vi "Firmware Manager.vi"() -> ()   [LabVIEW 2018]
uses:
  Type Defs/Firmware Action.ctl
  Type Defs/State Machine.ctl
panel:
  out "Wait":bool
  out "Error Out":errorcluster
  in  "Error In":errorcluster
  in  "Exit":bool
  in  "Start":bool
  out "Description":string
  in  "Firmware Backup Folder":path
  out "Messages":string
  in  "FW Action":T1
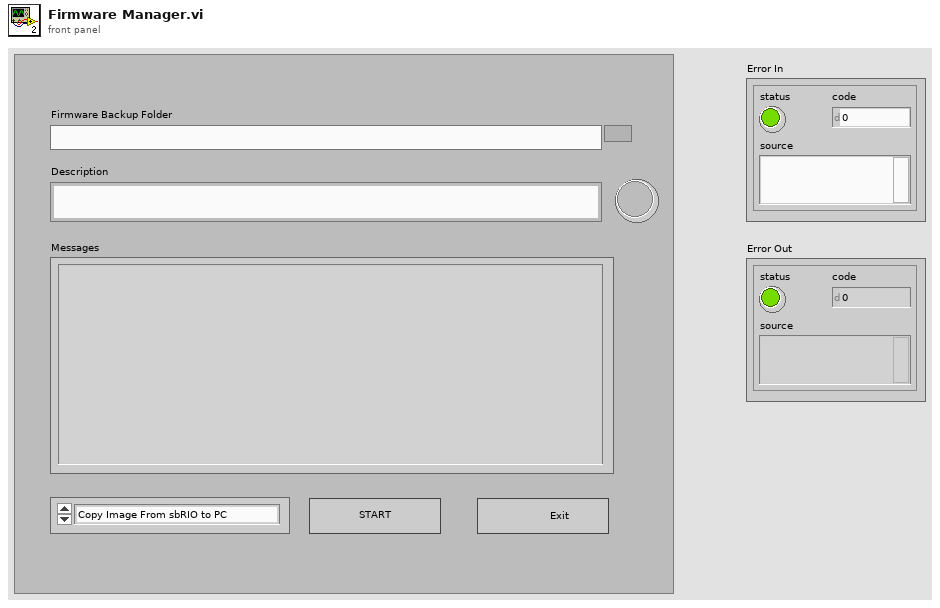
[diagram p1: front panel]
types:
  T1 = typedef "Firmware Action.ctl" = enum16{"Copy Image From sbRIO to PC", "Update Firmware From PC"}
  T2 = enum8{"Enabled", "Disabled", "Disabled and Grayed Out"}
  T3 = typedef "State Machine.ctl" = enum16{"Init", "Case 0", "Case 1", "Case 2", "Case 3", "Case 4", "Case 5", "Case 6", "Case 7", "Case 8", "Case 9", "Case 10", "Error", "Exit"}
  T4 = cluster{"Model":string, "MAC Address":string, "Hostname":string}
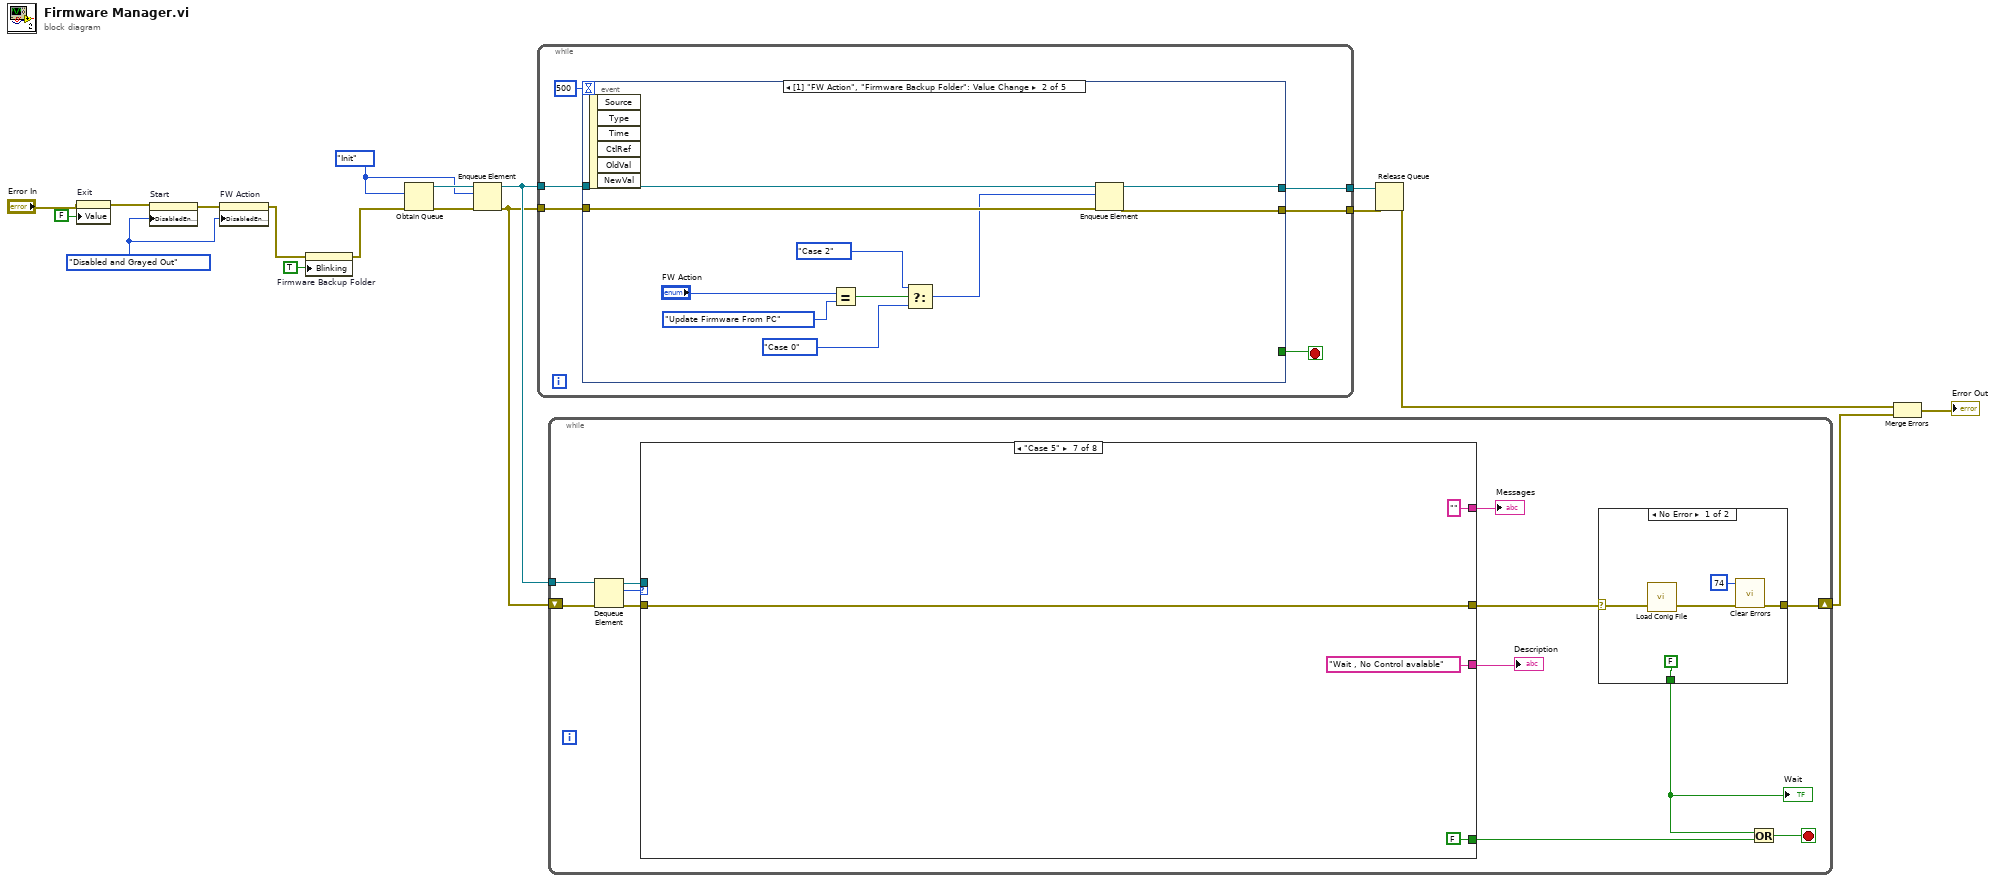
[diagram p0: block diagram]
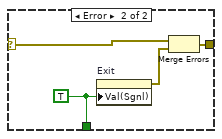
[diagram p2: hidden frame]
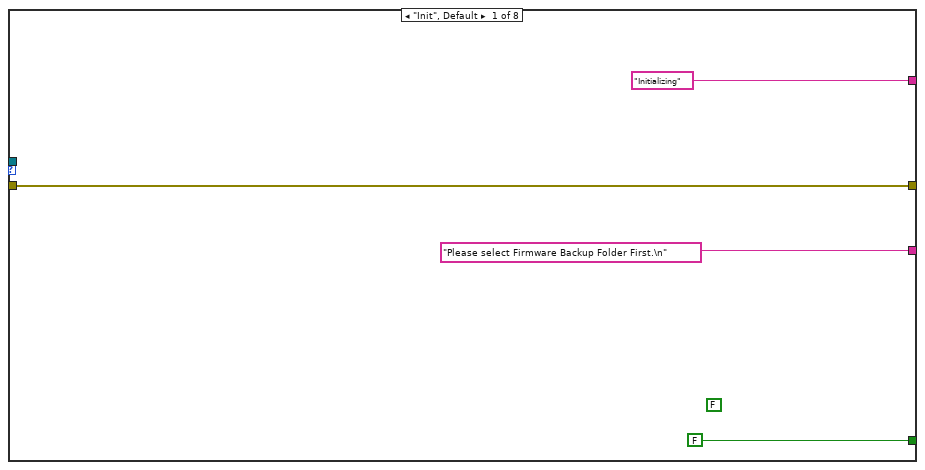
[diagram p3: hidden frame]
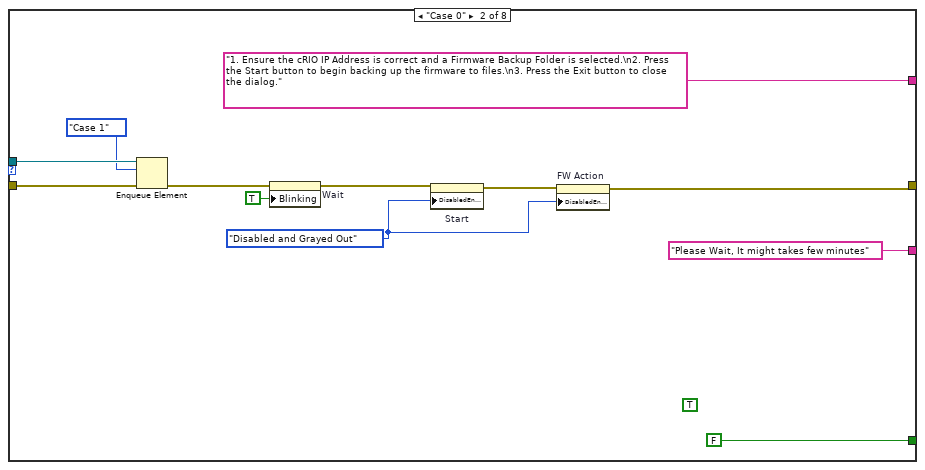
[diagram p4: hidden frame]
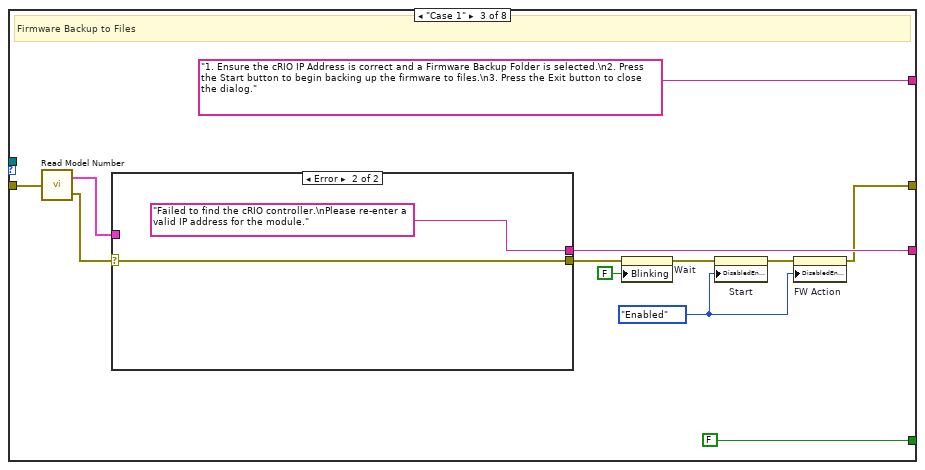
[diagram p5: hidden frame]
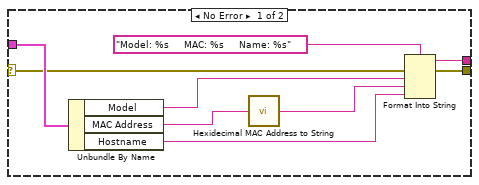
[diagram p6: hidden frame]
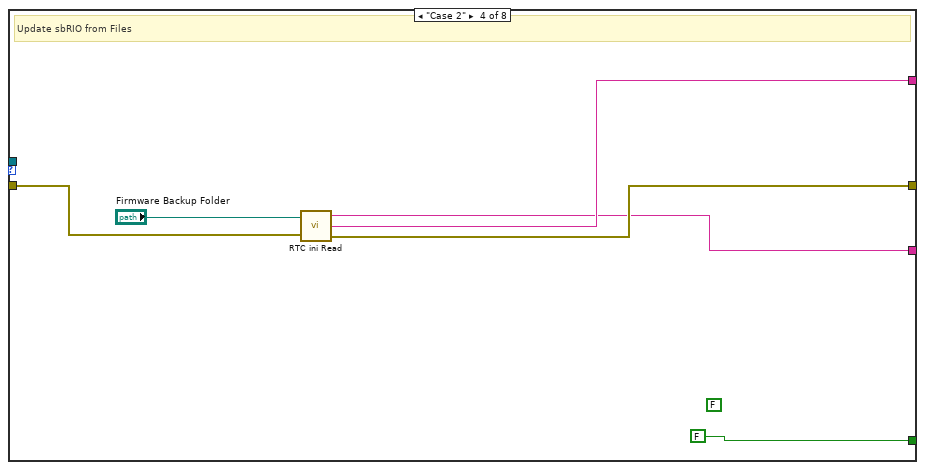
[diagram p7: hidden frame]
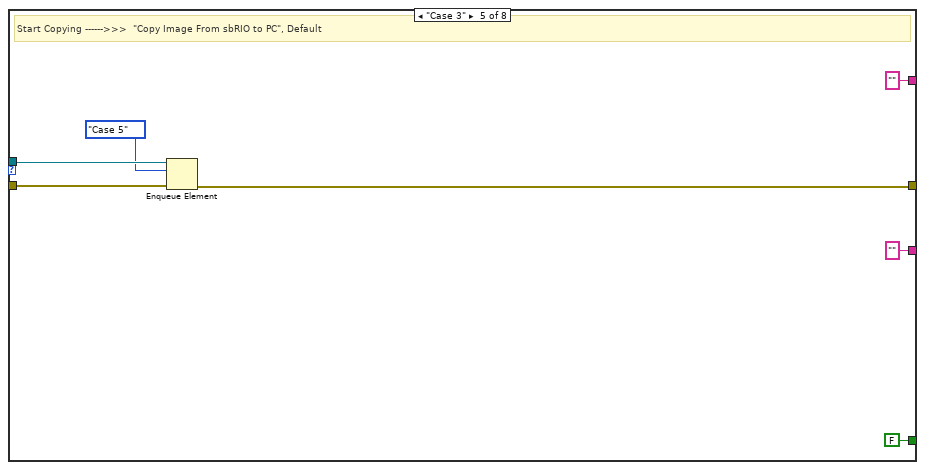
[diagram p8: hidden frame]
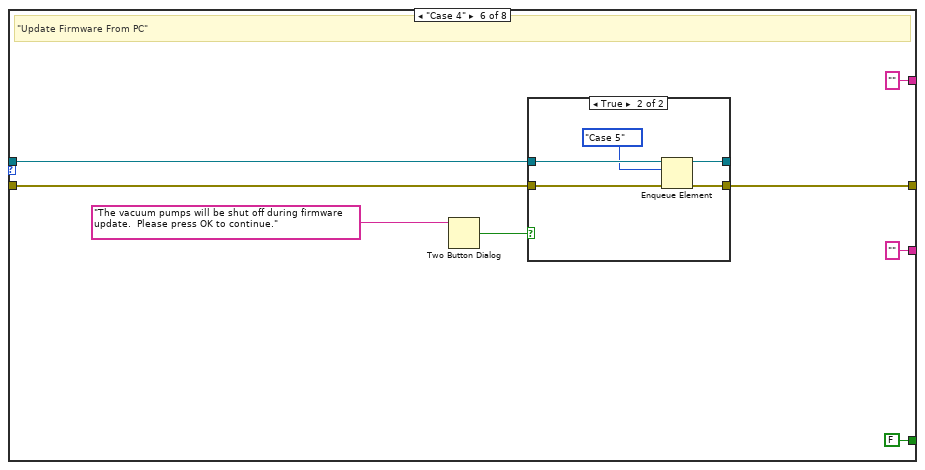
[diagram p9: hidden frame]
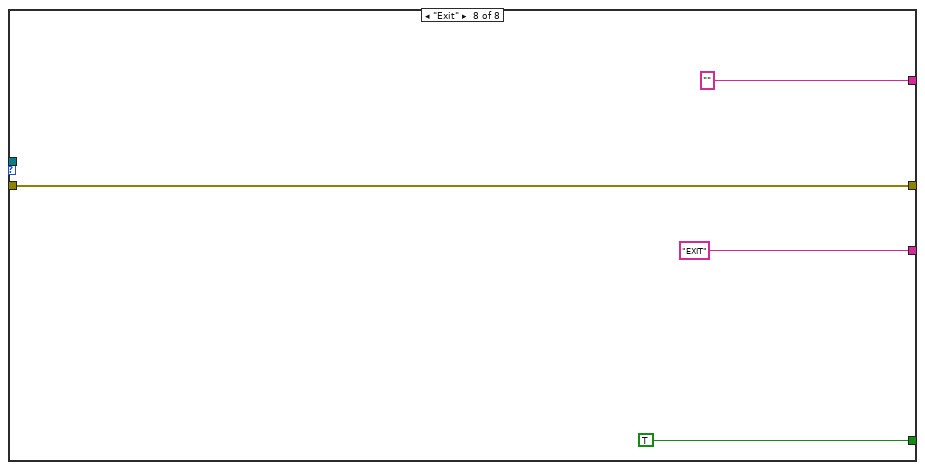
[diagram p11: hidden frame]
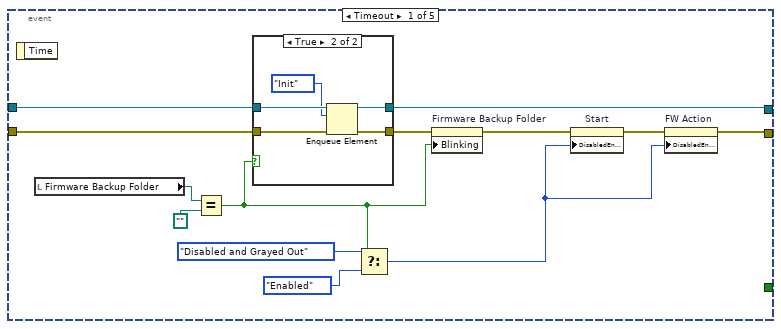
[diagram p12: hidden frame]
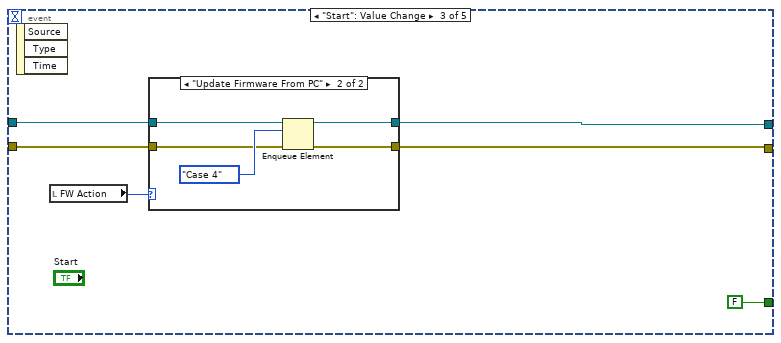
[diagram p14: hidden frame]
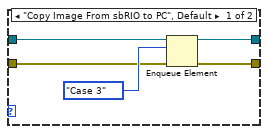
[diagram p15: hidden frame]
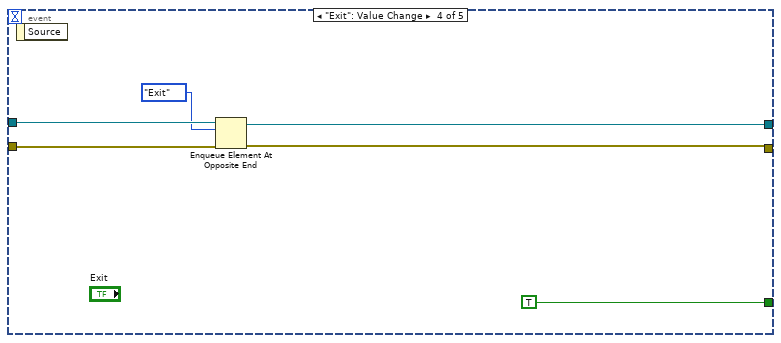
[diagram p16: hidden frame]
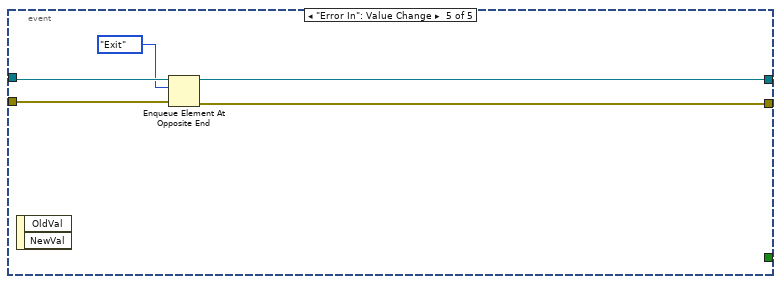
[diagram p17: hidden frame]
diagram:
  w4 = T2."Disabled and Grayed Out" ("Disabled")
  w16 = State_Machine."Init" ("Enum")
  n1 = property on="Exit" class="Bool (strict)"(error in="Error In", "Value"=FALSE ("Exit")) -> (error out=w6:errorcluster)  [unwired: 1 in, 1 out]
  n2 = property on="Start" class="Bool"(error in=w6, "DisabledEnum"=w4) -> (error out=w5:errorcluster)  [unwired: 1 in, 1 out]
  n3 = property on="FW Action" class="Enum (strict)"(error in=w5, "DisabledEnum"=w4) -> (error out=w3:errorcluster)  [unwired: 1 in, 1 out]
  n4 = property on="Firmware Backup Folder" class="Path"(error in=w3, "Blinking"=TRUE) -> (error out=w2:errorcluster)  [unwired: 1 in, 1 out]
  n5 = Obtain Queue(element data type=w16, error in (no error)=w2) -> (queue out=w18:refnum<queue>, error out=w17:errorcluster)  [unwired: 3 in, 1 out]
  n6 = Enqueue Element(queue=w18, element=w16, error in (no error)=w17) -> (queue out=w15:refnum<queue>, error out=w14:errorcluster)  [unwired: 1 in, 1 out]
  n7 = while {
    tunnel: w15 -> [w23]
    tunnel: w14 -> [w24]
    tunnel: [w20] -> w13
    tunnel: [w19] -> w10
    stop <- w22 stop-if-true
    n8 = event shown="[1] \"FW Action\", \"Firmware Backup Folder\": Value Change" {
      selector: _ -> [_ _ _ _ _]
      dyn-events: _ -> [_ _ _ _ _]
      timeout: 500 -> [_ _ _ _ _]
      tunnel: w24 -> [w28 w54 w58 w75 w81]
      tunnel: w23 -> [w27 w53 w57 w74 w80]
      tunnel: [_ _ FALSE TRUE _] -> w22
      tunnel: [w26 w52 w56 w71 w78] -> w19
      tunnel: [w34 w51 w55 w72 w77] -> w20
      event Timeout {
        n9 = event-data() -> ()  [unwired: 1 in, 1 out]
        n10 = local read "Firmware Backup Folder"() -> (w30:path)
        n11 = Equal?(x=w30, y=path "") -> (x = y?=w29:bool)
        n12 = case shown="True" w29 {
          tunnel: w28 -> [w38 w42]
          tunnel: w27 -> [w39 w44]
          tunnel: [w38 w41] -> w25
          tunnel: [w39 w40] -> w26
          frame False {
          }
          frame True {
            n13 = Enqueue Element(queue=w44, element=State_Machine."Init" ("Enum"), error in (no error)=w42) -> (queue out=w40:refnum<queue>, error out=w41:errorcluster)  [unwired: 1 in, 1 out]
          }
        }
        n14 = Select(t=T2."Disabled and Grayed Out" ("Disabled"), s=w29, f=T2."Enabled" ("Disabled")) -> (s? t:f=w32:T2)
        n15 = property on="Firmware Backup Folder" class="Path"(error in=w25, "Blinking"=w29) -> (error out=w31:errorcluster)  [unwired: 1 in, 1 out]
        n16 = property on="Start" class="Bool"(error in=w31, "DisabledEnum"=w32) -> (error out=w33:errorcluster)  [unwired: 1 in, 1 out]
        n17 = property on="FW Action" class="Enum (strict)"(error in=w33, "DisabledEnum"=w32) -> (error out=w34:errorcluster)  [unwired: 1 in, 1 out]
      }
      event "Firmware Backup Folder": Value Change {
        n18 = event-data() -> ()  [unwired: 1 in, 6 out]
        n19 = Equal?(x="FW Action", y=Firmware_Action."Update Firmware From PC" ("FW Action")) -> (x = y?=w48:bool)
        n20 = Select(t=State_Machine."Case 2" ("Enum"), s=w48, f=State_Machine."Case 0" ("Enum")) -> (s? t:f=w45:T3)
        n21 = Enqueue Element(queue=w53, element=w45, error in (no error)=w54) -> (queue out=w52:refnum<queue>, error out=w51:errorcluster)  [unwired: 1 in, 1 out]
      }
      event "Start": Value Change {
        n22 = event-data() -> ()  [unwired: 1 in, 3 out]
        n23 = local read "FW Action"() -> (w59:T1)
        n24 = case shown="\"Update Firmware From PC\"" w59 {
          tunnel: w58 -> [w64 w69]
          tunnel: w57 -> [w63 w68]
          tunnel: [w62 w67] -> w55
          tunnel: [w61 w66] -> w56
          frame "Copy Image From sbRIO to PC", Default {
            n25 = Enqueue Element(queue=w63, element=State_Machine."Case 3" ("Enum"), error in (no error)=w64) -> (queue out=w61:refnum<queue>, error out=w62:errorcluster)  [unwired: 1 in, 1 out]
          }
          frame "Update Firmware From PC" {
            n26 = Enqueue Element(queue=w68, element=State_Machine."Case 4" ("Enum"), error in (no error)=w69) -> (queue out=w66:refnum<queue>, error out=w67:errorcluster)  [unwired: 1 in, 1 out]
          }
        }
      }
      event "Exit": Value Change {
        n27 = event-data() -> ()  [unwired: 1 in, 1 out]
        n28 = Enqueue Element At Opposite End(queue=w74, element=State_Machine."Exit" ("Enum"), error in (no error)=w75) -> (queue out=w71:refnum<queue>, error out=w72:errorcluster)  [unwired: 1 in, 1 out]
      }
      event "Error In": Value Change {
        n29 = event-data() -> ()  [unwired: 1 in, 2 out]
        n30 = Enqueue Element At Opposite End(queue=w80, element=State_Machine."Exit" ("Enum"), error in (no error)=w81) -> (queue out=w78:refnum<queue>, error out=w77:errorcluster)  [unwired: 1 in, 1 out]
      }
    }
  }
  n31 = while {
    tunnel: w15 -> [w93]
    shift-right: [w85] -> w12
    shift-left: w14 -> [w92]
    stop <- w87 stop-if-true
    n32 = Dequeue Element(queue=w93, error in (no error)=w92) -> (queue out=w90:refnum<queue>, element=w91:T3, error out=w89:errorcluster)  [unwired: 1 in, 1 out]
    n33 = case shown="\"Case 5\"" w91 {
      tunnel: w90 -> [_ w114 _ _ w153 w160 _ _]
      tunnel: w89 -> [w105 w115 w128 w145 w154 w161 w173 w177]
      tunnel: [w105 w108 w121 w144 w151 w158 w173 w177] -> w88
      tunnel: [FALSE FALSE FALSE FALSE FALSE FALSE FALSE TRUE] -> w86
      tunnel: ["Initializing" ("t") "1. Ensure the cRIO IP Address is correct and a Firmware Backup Folder is selected.\n2. Press the Start button to begin backing up the firmware to files.\n3. Press the Exit button to close the dialog." ("t") "1. Ensure the cRIO IP Address is correct and a Firmware Backup Folder is selected.\n2. Press the Start button to begin backing up the firmware to files.\n3. Press the Exit button to close the dialog." ("t") w143 "" ("t") "" ("t") "" ("t") "" ("t")] -> w84
      tunnel: ["Please select Firmware Backup Folder First.\n" ("t") "Please Wait, It might takes few minutes" ("t") w125 w142 "" ("t") "" ("t") "Wait , No Control avalable" ("t") "EXIT" ("t")] -> w83
      frame "Init", Default {
        (unwired) FALSE
      }
      frame "Case 0" {
        w107 = T2."Disabled and Grayed Out" ("Disabled")
        (unwired) TRUE
        n34 = Enqueue Element(queue=w114, element=State_Machine."Case 1" ("Enum"), error in (no error)=w115) -> (error out=w112:errorcluster)  [unwired: 1 in, 2 out]
        n35 = property on="Wait" class="Bool (strict)"(error in=w112, "Blinking"=TRUE) -> (error out=w110:errorcluster)  [unwired: 1 in, 1 out]
        n36 = property on="Start" class="Bool"(error in=w110, "DisabledEnum"=w107) -> (error out=w109:errorcluster)  [unwired: 1 in, 1 out]
        n37 = property on="FW Action" class="Enum (strict)"(error in=w109, "DisabledEnum"=w107) -> (error out=w108:errorcluster)  [unwired: 1 in, 1 out]
      }
      frame "Case 1" {
        w120 = T2."Enabled" ("Disabled")
        # "Firmware Backup to Files"
        n38 = call "Read Model Number.vi"("Error In"=w128) -> ("Target Info"=w126:T4, "Error Out"=w127:errorcluster)
        n39 = case shown="Error" w127 {
          selector: w127 -> [w137 w141]
          tunnel: w126 -> [w139 _]
          tunnel: [w132 "Failed to find the cRIO controller.\nPlease re-enter a valid IP address for the module." ("t")] -> w125
          tunnel: [w131 w141] -> w124
          frame No Error {
            n40 = Unbundle By Name(w139) -> ("Model"=w136:string, "MAC Address"=w135:string, "Hostname"=w134:string)
            n41 = call "Hexidecimal MAC Address to String.vi"("MAC Address"=w135) -> ("MAC Address ("=w133:string)
            n42 = Format Into String(format string="Model: %s     MAC: %s     Name: %s", error in=w137, w136, w133, w134) -> (resulting string=w132:string, error out=w131:errorcluster)  [unwired: 1 in]
          }
          frame Error {
          }
        }
        n43 = property on="Wait" class="Bool (strict)"(error in=w124, "Blinking"=FALSE) -> (error out=w122:errorcluster)  [unwired: 1 in, 1 out]
        n44 = property on="Start" class="Bool"(error in=w122, "DisabledEnum"=w120) -> (error out=w119:errorcluster)  [unwired: 1 in, 1 out]
        n45 = property on="FW Action" class="Enum (strict)"(error in=w119, "DisabledEnum"=w120) -> (error out=w121:errorcluster)  [unwired: 1 in, 1 out]
      }
      frame "Case 2" {
        (unwired) FALSE
        # "Update sbRIO from Files"
        n46 = call "RTC ini Read.vi"("Firmware Backup Folder"="Firmware Backup Folder", "error in (no error)"=w145) -> ("Description"=w142:string, "Messages"=w143:string, "error out"=w144:errorcluster)
      }
      frame "Case 3" {
        # "Start Copying ------>>>  \"Copy Image From sbRIO to PC\", Default"
        n47 = Enqueue Element(queue=w153, element=State_Machine."Case 5" ("Enum"), error in (no error)=w154) -> (error out=w151:errorcluster)  [unwired: 1 in, 2 out]
      }
      frame "Case 4" {
        # "\"Update Firmware From PC\""
        n48 = Two Button Dialog(message="The vacuum pumps will be shut off during firmware update.  Please press OK to continue.") -> (T button?=w159:bool)  [unwired: 2 out]
        n49 = case shown="True" w159 {
          tunnel: w161 -> [w163 w168]
          tunnel: w160 -> [w164 w169]
          tunnel: [w164 w167] -> _
          tunnel: [w163 w166] -> w158
          frame False {
          }
          frame True {
            n50 = Enqueue Element(queue=w169, element=State_Machine."Case 5" ("Enum"), error in (no error)=w168) -> (queue out=w167:refnum<queue>, error out=w166:errorcluster)  [unwired: 1 in, 1 out]
          }
        }
      }
      frame "Case 5" {
      }
      frame "Exit" {
      }
    }
    "Messages" <- w84
    "Description" <- w83
    n51 = case shown="No Error" w88 {
      selector: w88 -> [w97 w100]
      tunnel: [FALSE w102] -> w82
      tunnel: [w95 w101] -> w85
      frame No Error {
        n52 = call "Load Conig File.vi"("error in (no error)"=w97) -> ("error out"=w96:errorcluster)  [unwired: 1 in, 1 out]
        n53 = call <vilib>:"Clear Errors.vi"("error in (no error)"=w96, "specific error code to clear (0: all)"=74) -> ("error out"=w95:errorcluster)  [unwired: 4 in, 1 out]
      }
      frame Error {
        w102 = TRUE ("Exit")
        n54 = property on="Exit" class="Bool (strict)"("Val(Sgnl)"=w102) -> (error out=w99:errorcluster)  [unwired: 2 in, 1 out]
        n55 = Merge Errors(w100, w99) -> (w101:errorcluster)
      }
    }
    "Wait" <- w82
    n56 = Or(x=w82, y=w86) -> (x .or. y?=w87:bool)
  }
  n57 = Release Queue(queue=w10, error in (no error)=w13) -> (error out=w8:errorcluster)  [unwired: 1 in, 2 out]
  n58 = Merge Errors(w8, w12) -> (→"Error Out":errorcluster)
